vi "AO to Channel.vi"(10 "Analog Output":T1) -> (2 "Channel":i32)   [LabVIEW 2020, in "HandsOnPi2040.lvlib"]
doc: "Converts an Analog Output into the required channel."
uses:
  HandsOnPi2040.lvlib
  Public/AOs.ctl
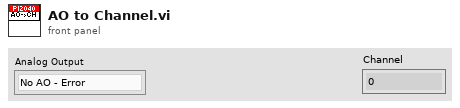
[diagram p1: front panel]
types:
  T1 = typedef "HandsOnPi2040.lvlib/AOs.ctl" = enum8{"No AO - Error", "AO1"}
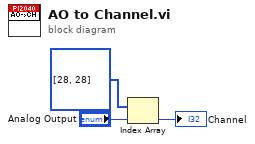
[diagram p0: block diagram]
diagram:
  n1 = Index Array(array=i32[] [28, 28], index="Analog Output") -> (element=→"Channel":i32)
